vi "Circular.vi"   [LabVIEW 2016]
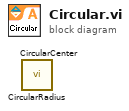
[diagram p0: block diagram]
diagram:
  n1 = call "CircularRadius.vi"() -> ()  [unwired: 18 in, 2 out]
  n2 = call "CircularCenter.vi"() -> ()  [unwired: 18 in, 2 out]
